vi "example_move_motor_to_position_with_status.vi"() -> ()   [LabVIEW 2012]
doc: "EXAMPLE: Move To Target (with status)\n\nThis example VI moves the motor to a desired target position while displaying the current runtime status. If that position should exceed the counter limitations of the motor, an error will be triggered and the move will not take place.\n\nFurthermore, the VI issues an enable command before attempting the move (to be sure the motor is actually ready to move).\n\nProduced By:\n\nChristopher Lemieux\nKod Integrations, LLC\n4835 Marianne Drive\nMount Airy, MD 21771\nhttp://www.kodintegrations.com\nemail: clemieux@kodintegrations.com\nphone: (240) 687-1288"
uses:
  utilities/getters/controls/status_states.ctl
  main_functions/commands.ctl
panel:
  out "other_states":T1[](array[typedef])
  out "motion_state":T1=enum."CONST"
  in  "stop":bool
  in  "New Position:":i32
  in  "device_index (def=0)":i32
  out "error out":errorcluster
  in  "error in (no error)":errorcluster
  # "To Operate:\n\n(1) Enter the Device Index. If only one is connected\nthen leave as the default (0)\n\n(2) Enter the new position to move the motor to.  Be sure\nit's not the same position where the motor currently sits\n\n(3) click the arrow button to run the VI\n\n(4) note the change in misc device states while the motor\nruns\n\n(5) click the STOP button to properly terminate connection\nwith the device"
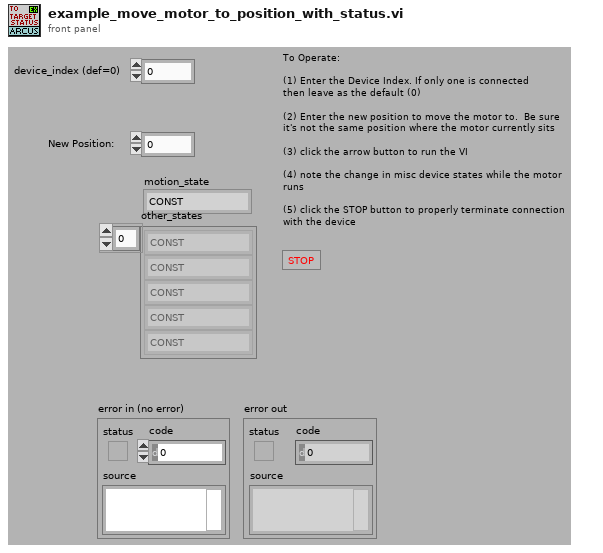
[diagram p1: front panel]
types:
  T1 = typedef "status_states.ctl" = enum16{"IDLE", "CONST", "ACCEL", "DECEL", "HOME_SWITCH", "-LIMIT_SWITCH", "+LIMIT_SWITCH", "-LIMIT_ERR", "+LIMIT_ERR", "COMM_ERR"}
  T2 = typedef "commands.ctl" = enum16{"clearErr", "constJogNeg", "constJogPos", "getAccel", "getActualAmp", "getDeviceId", "getDigInputStatus", "getDigInputsStatus", "getDigOutputStatus", "getDigOutputsStatus", "getFirmwareVer", "getHighSpeed", "getIdleAmp", "getLowSpeed", "getMicroStep", "getMotorStatus", "getMoveMode", "getPolarity", "getPosition", "getProdId", "getPwrStatus", "getRunAmp", "getStatus", "homeNeg", "homePos", "moveToPosition", "powerDown", "powerUp", "setAccel", "setDeviceId", "setDigOutput", "setDigOutputs", "setHighSpeed", "setIdleAmp", "setLowSpeed", "setMoveModeAbs", "setMoveModeIncr", "setPolarity", "setPosition", "setRunAmp", "stopNow", "stopSlow", "storeToMem"}
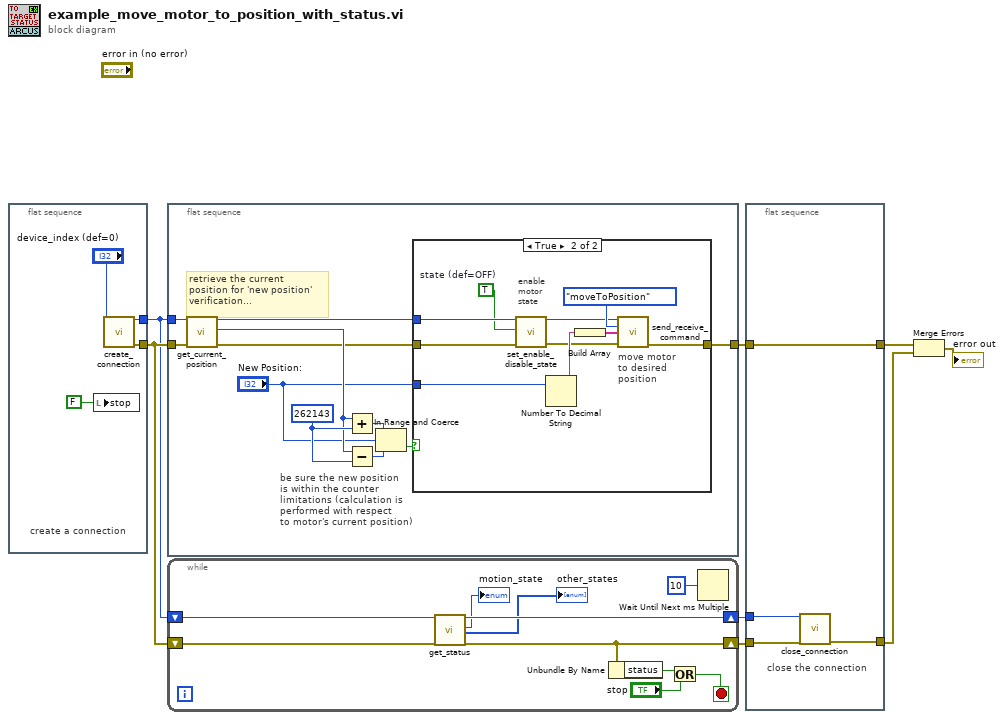
[diagram p0: block diagram]
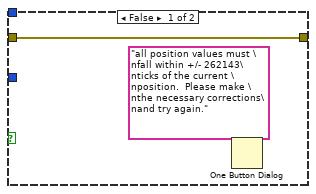
[diagram p2: hidden frame]
diagram:
  n1 = flat-sequence {
    tunnel: [w11] -> w4
    tunnel: [w10] -> w8
    frame #0 {
      # "create a connection"
      n2 = local write "stop"(FALSE ("stop")) -> ()
      n3 = call "create_connection.vi"("device_index (def=0)"="device_index (def=0)") -> ("reference"=w11:i32, "error out"=w10:errorcluster)  [unwired: 13 in]
    }
  }
  n4 = flat-sequence {
    tunnel: w4 -> [w23]
    tunnel: w8 -> [w22]
    tunnel: [w13] -> w7
    frame #0 {
      w19 = 262143
      # "retrieve the current\nposition for 'new position'\nverification..."
      # "be sure the new position\nis within the counter \nlimitations (calculation is\nperformed with respect\nto motor's current position)"
      n5 = call "get_current_position.vi"("reference (in)"=w23, "error in (no error)"=w22) -> ("reference (dup)"=w15:i32, "current_position (units)"=w18:i32, "error out"=w17:errorcluster)  [unwired: 15 in]
      n6 = Add(x=w18, y=w19) -> (x+y=w21:i32)
      n7 = Subtract(x=w18, y=w19) -> (x-y=w20:i32)
      n8 = In Range and Coerce(upper limit=w21, x="New Position:", lower limit=w20) -> (In Range?=w16:bool)  [unwired: 1 out]
      n9 = case shown="True" w16 {
        tunnel: w17 -> [w25 w30]
        tunnel: [w25 w26] -> w13
        tunnel: w15 -> [_ w31]
        tunnel: "New Position:" -> [_ w34]
        frame False {
          n10 = One Button Dialog(message="all position values must \nfall within +/- 262143\nticks of the current \nposition.  Please make \nthe necessary corrections\nand try again.") -> ()  [unwired: 1 in, 1 out]
        }
        frame True {
          w29 = TRUE  # state (def=OFF)
          # "move motor\nto desired\nposition"
          # "enable\nmotor\nstate"
          n11 = call "set_enable_disable_state.vi"("reference (in)"=w31, "state (def=OFF)"=w29, "error in (no error)"=w30) -> ("reference (dup)"=w27:i32, "error out"=w28:errorcluster)  [unwired: 14 in, 1 out]
          n12 = Number To Decimal String(number=w34) -> (decimal integer string=w33:string)  [unwired: 1 in]
          n13 = Build Array(w33) -> (w32:string[])
          n14 = call "send_receive_command.vi"("reference (in)"=w27, "command"=commands."moveToPosition", "params (opt)"=w32, "error in (no error)"=w28) -> ("error out"=w26:errorcluster)  [unwired: 7 in, 4 out]
        }
      }
    }
  }
  n15 = while {
    shift-right: [w44] -> w2
    shift-left: w8 -> [w45]
    shift-right: [w39] -> w3
    shift-left: w4 -> [w40]
    stop <- w42 stop-if-true
    n16 = call "get_status.vi"("reference (in)"=w40, "error in (no error)"=w45) -> ("reference (dup)"=w39:i32, "motion_state"=→"motion_state":T1, "other_states"=→"other_states":T1[], "error out"=w44:errorcluster)  [unwired: 13 in, 1 out]
    n17 = Unbundle By Name(w44) -> ("status"=w43:bool)
    n18 = Or(x=w43, y="stop") -> (x .or. y?=w42:bool)
    n19 = Wait Until Next ms Multiple(millisecond multiple=u32 10) -> ()  [unwired: 1 out]
  }
  n20 = flat-sequence {
    tunnel: w7 -> [w47]
    tunnel: [w47] -> w6
    tunnel: w3 -> [w49]
    tunnel: w2 -> [w48]
    tunnel: [w46] -> w1
    frame #0 {
      # "close the connection"
      n21 = call "close_connection.vi"("reference"=w49, "error in (no error)"=w48) -> ("error out"=w46:errorcluster)  [unwired: 13 in]
    }
  }
  n22 = Merge Errors(w6, w1) -> (→"error out":errorcluster)
